vi "process_mul_div.vi"(11 "expression":string) -> (1 "position":u16, 2 "value":dbl)   [LabVIEW 2021]
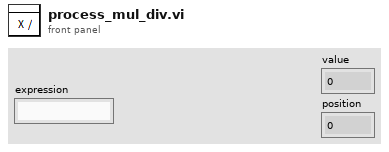
[diagram p1: front panel]
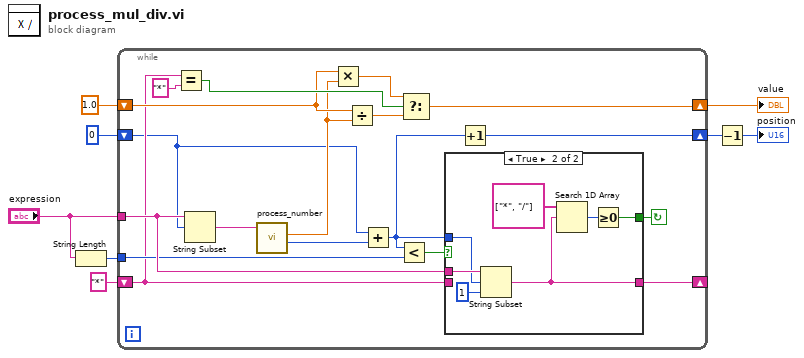
[diagram p0: block diagram]
diagram:
  n1 = String Length(string="expression") -> (length=w5:i32)
  n2 = while {
    tunnel: w5 -> [w19]
    shift-right: [w20] -> w1
    shift-left: 1.0 -> [w22]
    shift-right: [w16] -> w3
    shift-left: u16 0 ("position") -> [w9]
    tunnel: "expression" -> [w26]
    shift-right: [w14] -> _
    shift-left: "*" -> [w13]
    stop <- w15 continue-if-true
    n3 = Equal?(x=w13, y="*") -> (x = y?=w24:bool)
    n4 = String Subset(string=w26, offset (0)=w9) -> (substring=w12:string)  [unwired: 1 in]
    n5 = call "process_number.vi"("expression"=w12) -> ("position"=w10:u16, "value"=w11:dbl)  [unwired: 9 in]
    n6 = Multiply(x=w22, y=w11) -> (x*y=w23:dbl)
    n7 = Divide(x=w22, y=w11) -> (x/y=w21:dbl)
    n8 = Add(x=w9, y=w10) -> (x+y=w17:u16)
    n9 = Less?(x=w17, y=w19) -> (x < y?=w18:bool)
    n10 = Select(t=w23, s=w24, f=w21) -> (s? t:f=w20:dbl)
    n11 = case shown="True" w18 {
      selector: w18 -> [w28 _]
      tunnel: w26 -> [_ w32]
      tunnel: w17 -> [_ w31]
      tunnel: [w28 w33] -> w15
      tunnel: [w27 w29] -> w14
      tunnel: w13 -> [w27 _]
      frame False {
      }
      frame True {
        n12 = String Subset(string=w32, offset (0)=w31, length (rest)=1 ("length (rest)")) -> (substring=w29:string)
        n13 = Search 1D Array(1D array=string[] ["*", "/"], element=w29) -> (index of element=w34:i32)  [unwired: 1 in]
        n14 = Greater Or Equal To 0?(x=w34) -> (x >= 0?=w33:bool)
      }
    }
    n15 = Increment(x=w17) -> (x+1=w16:u16)
  }
  "value" <- w1
  n16 = Decrement(x=w3) -> (x-1=→"position":u16)
